vi "Serial Read.vi"(8 "error in":errorcluster, 9 "timeout (ms)":i32, 10 "bytes to read":i32, 11 "Visa Resource":refnum<visa-resource-name>) -> (0 "error out":errorcluster, 1 "timed out?":bool, 3 "data":u8[](array[numeric]))   [LabVIEW 2014, in "MyLib.lvlib" / "Serial Shared Components.lvlib"]
doc: "Performs a read on the serial port."
uses:
  Serial Shared Components.lvlib
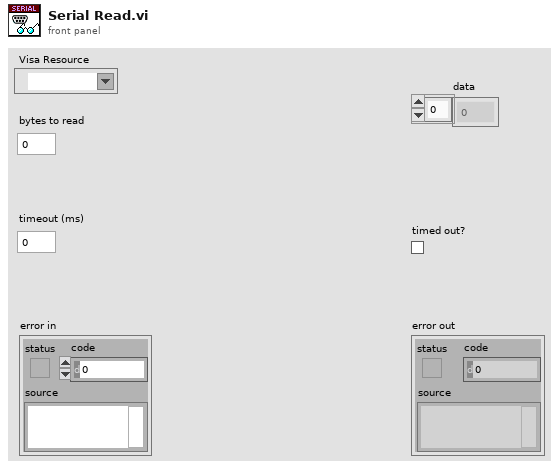
[diagram p1: front panel]
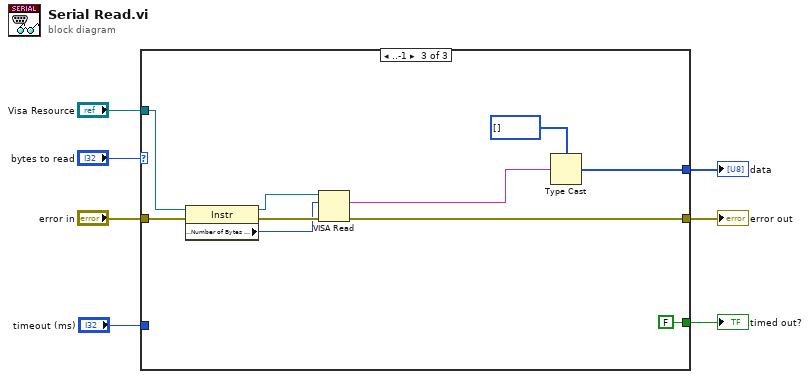
[diagram p0: block diagram]
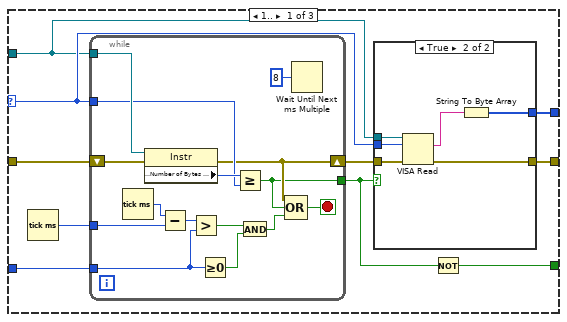
[diagram p2: hidden frame]
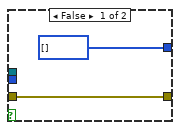
[diagram p3: hidden frame]
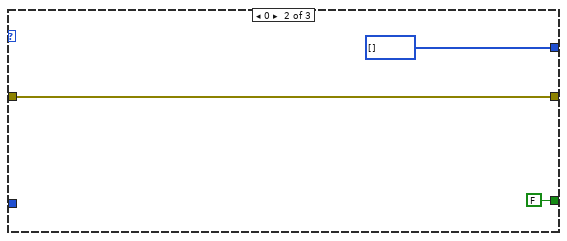
[diagram p4: hidden frame]
diagram:
  n1 = case shown="..-1" "bytes to read" {
    selector: "bytes to read" -> [w12 _ _]
    tunnel: "timeout (ms)" -> [w10 _ _]
    tunnel: "error in" -> [w16 w43 w53]
    tunnel: "Visa Resource" -> [w11 _ w52]
    tunnel: [w14 w43 w48] -> w2
    tunnel: [w13 u8[] [] ("data") w46] -> w3
    tunnel: [w8 FALSE FALSE] -> w1
    frame 1.. {
      n2 = Tick Count (ms)() -> (millisecond timer value=w17:u32)
      n3 = while {
        tunnel: w17 -> [w32]
        shift-right: [w36] -> w15
        shift-left: w16 -> [w40]
        tunnel: w12 -> [w37]
        tunnel: w11 -> [w39]
        tunnel: [w35] -> w9
        tunnel: w10 -> [w28]
        stop <- w34 stop-if-true
        n4 = Tick Count (ms)() -> (millisecond timer value=w33:u32)
        n5 = property class="Instr"(reference=w39, error in=w40) -> (error out=w36:errorcluster, "Serial Settings:Number of Bytes at Serial Port"=w38:u32)  [unwired: 1 out]
        n6 = Subtract(x=w33, y=w32) -> (x-y=w30:u32)
        n7 = Greater?(x=w30, y=w28) -> (0:w29:bool)
        n8 = Greater Or Equal To 0?(x=w28) -> (x >= 0?=w27:bool)
        n9 = Greater Or Equal?(x=w38, y=w37) -> (x >= y?=w35:bool)
        n10 = And(x=w29, y=w27) -> (x .and. y?=w31:bool)
        n11 = Compound Arithmetic op=OR(w36, w35, w31) -> (w34:bool)
        n12 = Wait Until Next ms Multiple(millisecond multiple=u32 8) -> ()  [unwired: 1 out]
      }
      n13 = case shown="True" w9 {
        tunnel: w11 -> [_ w23]
        tunnel: w15 -> [w18 w25]
        tunnel: [w18 w24] -> w14
        tunnel: [u8[] [] ("data") w21] -> w13
        tunnel: w12 -> [_ w22]
        frame False {
        }
        frame True {
          n14 = VISA Read(VISA resource name=w23, byte count=w22, error in (no error)=w25) -> (read buffer=w20:string, error out=w24:errorcluster)  [unwired: 2 out]
          n15 = String To Byte Array(string=w20) -> (unsigned byte array=w21:u8[])
        }
      }
      n16 = Not(x=w9) -> (.not. x?=w8:bool)
    }
    frame 0 {
    }
    frame ..-1 {
      n17 = property class="Instr"(reference=w52, error in=w53) -> (reference out=w50:refnum<visa-resource-name>, error out=w51:errorcluster, "Serial Settings:Number of Bytes at Serial Port"=w49:u32)
      n18 = VISA Read(VISA resource name=w50, byte count=w49, error in (no error)=w51) -> (read buffer=w45:string, error out=w48:errorcluster)  [unwired: 2 out]
      n19 = Type Cast(type=u8[] [] ("data"), x=w45) -> (*(type *) &x=w46:u8[])
    }
  }
  "error out" <- w2
  "data" <- w3
  "timed out?" <- w1
